vi "FTW-ERR-StatusCode.vi"(1 "error to check":errorcluster) -> (0 "Code":i32)   [LabVIEW 2013]
panel:
  # "Inputs"
  # "Outputs"
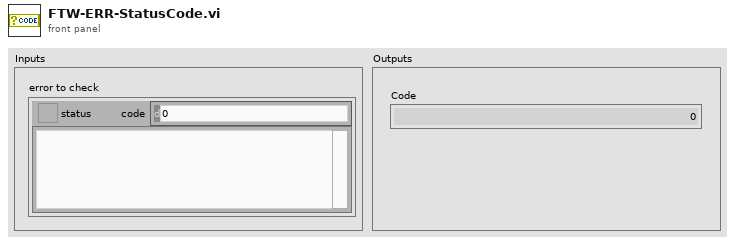
[diagram p1: front panel]
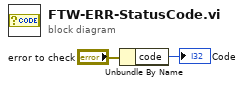
[diagram p0: block diagram]
diagram:
  n1 = Unbundle By Name("error to check") -> ("code"=→"Code":i32)
